vi "UpdateAWGGraph.vi"(9 "RF Sequence array":T1[](array[typedef]), 10 "MW sequence array":T1[](array[typedef]), 11 "Waveform Graph 2":refnum<vi>) -> ()   [LabVIEW 2019]
uses:
  controls/AWGpulse.ctl
  controls/AWGchannelcontrol.ctl
  <vilib>/measure/NI_MAPro.lvlib
panel:
  # "Name :"
  # "Timing :"
  # "Detuning :"
  # "Step :"
  # "Frequency :"
  # "Step :"
  # "Amplitude :"
  # "Step :"
  # "Phase  :"
  # "Step :"
  # "Name :"
  # "Timing :"
  # "Detuning :"
  # "Step :"
  # "Frequency :"
  # "Step :"
  # "Amplitude :"
  # "Step :"
  # "Phase  :"
  # "Step :"
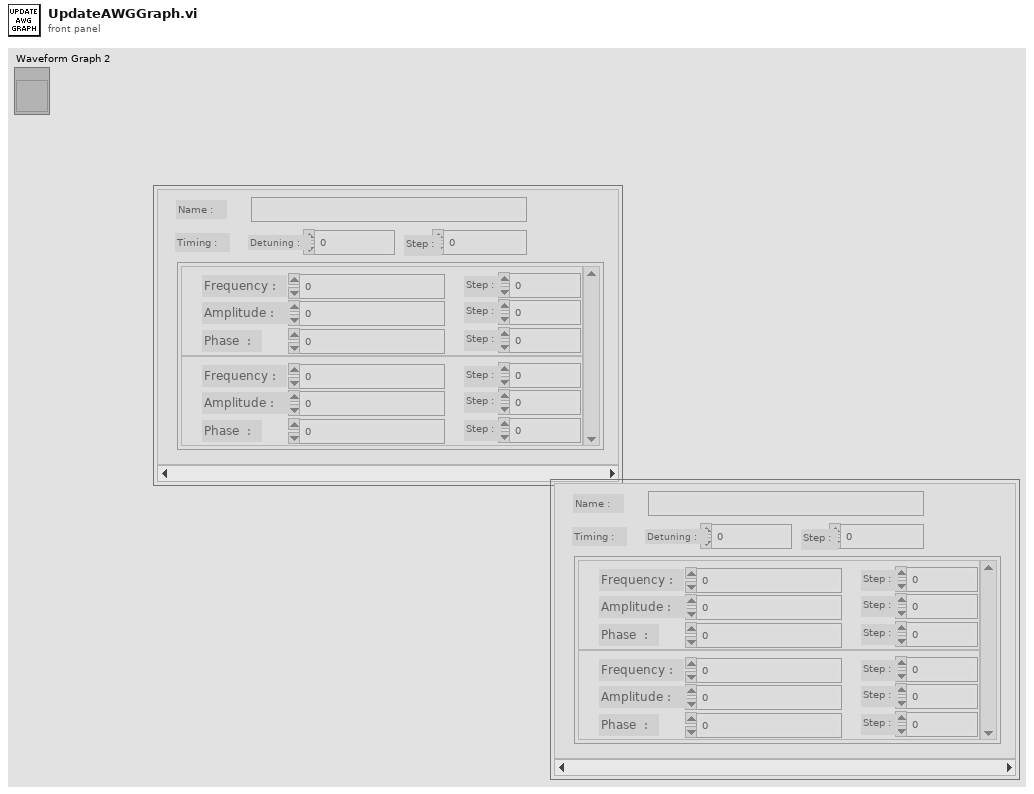
[diagram p1: front panel]
types:
  T1 = typedef "AWGpulse.ctl" = cluster{"Name":string, "time det":dbl, "time step":dbl, "Channel Array":T2[]}
  T2 = typedef "AWGchannelcontrol.ctl" = cluster{"freq\n":dbl, "freq step":dbl, "amp det":dbl, "amp step":dbl, "phase det":dbl, "phase step":dbl}
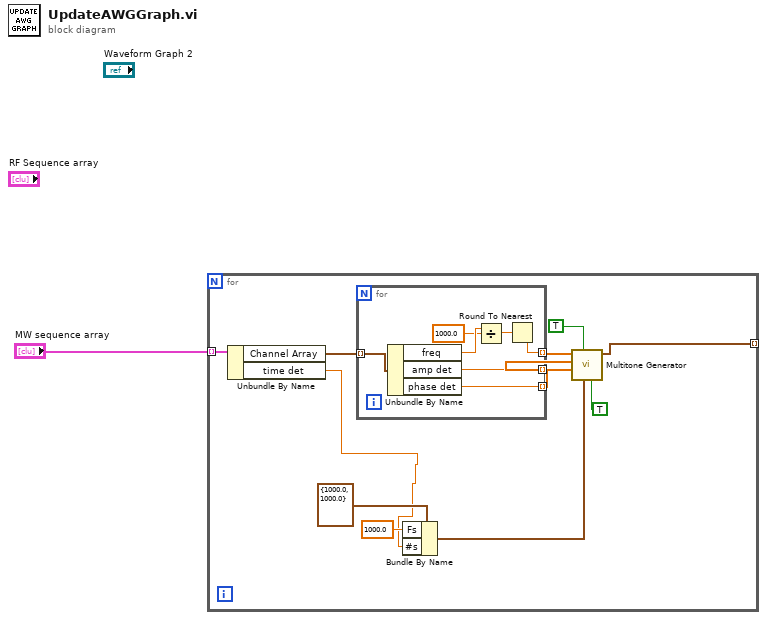
[diagram p0: block diagram]
diagram:
  n1 = for {
    tunnel: "MW sequence array" -> [w13] mode=indexing
    tunnel: [w2] -> _ mode=indexing
    n2 = Unbundle By Name(w13) -> ("Channel Array"=w12:T2[], "time det"=w4:dbl)
    n3 = for {
      tunnel: w12 -> [w20] mode=indexing
      tunnel: [w14] -> w11 mode=indexing
      tunnel: [w19] -> w10 mode=indexing
      tunnel: [w18] -> w9 mode=indexing
      n4 = Unbundle By Name(w20) -> ("freq"=w17:dbl, "amp det"=w19:dbl, "phase det"=w18:dbl)
      n5 = Divide(x=w17, y=1000.0) -> (x/y=w15:dbl)
      n6 = Round To Nearest(number=w15) -> (nearest integer value=w14:dbl)
    }
    n7 = Bundle By Name(cluster=cluster{"Fs":dbl, "#s":dbl} {"Fs"=1000.0, "#s"=1000.0} ("sampling info"), "Fs"=1000.0, "#s"=w4) -> (w5:cluster{"Fs":dbl, "#s":dbl})
    n8 = call <vilib>:"Multitone Generator.vi"("coerce frequencies?"=TRUE, "sampling info"=w5, "reset signal"=TRUE, "tone phases"=w9, "tone amplitudes"=w10, "tone frequencies"=w11) -> ("signal out"=w2:waveform(dbl))  [unwired: 2 in, 3 out]
  }
